vi "SALVAR.vi"() -> ()   [LabVIEW 2014]
uses:
  Global 5.vi
  Global 2.vi
  <vilib>/Utility/file.llb/Write To Spreadsheet File (DBL).vi
panel:
  out "Elapsed Time (s)":dbl
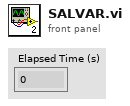
[diagram p1: front panel]
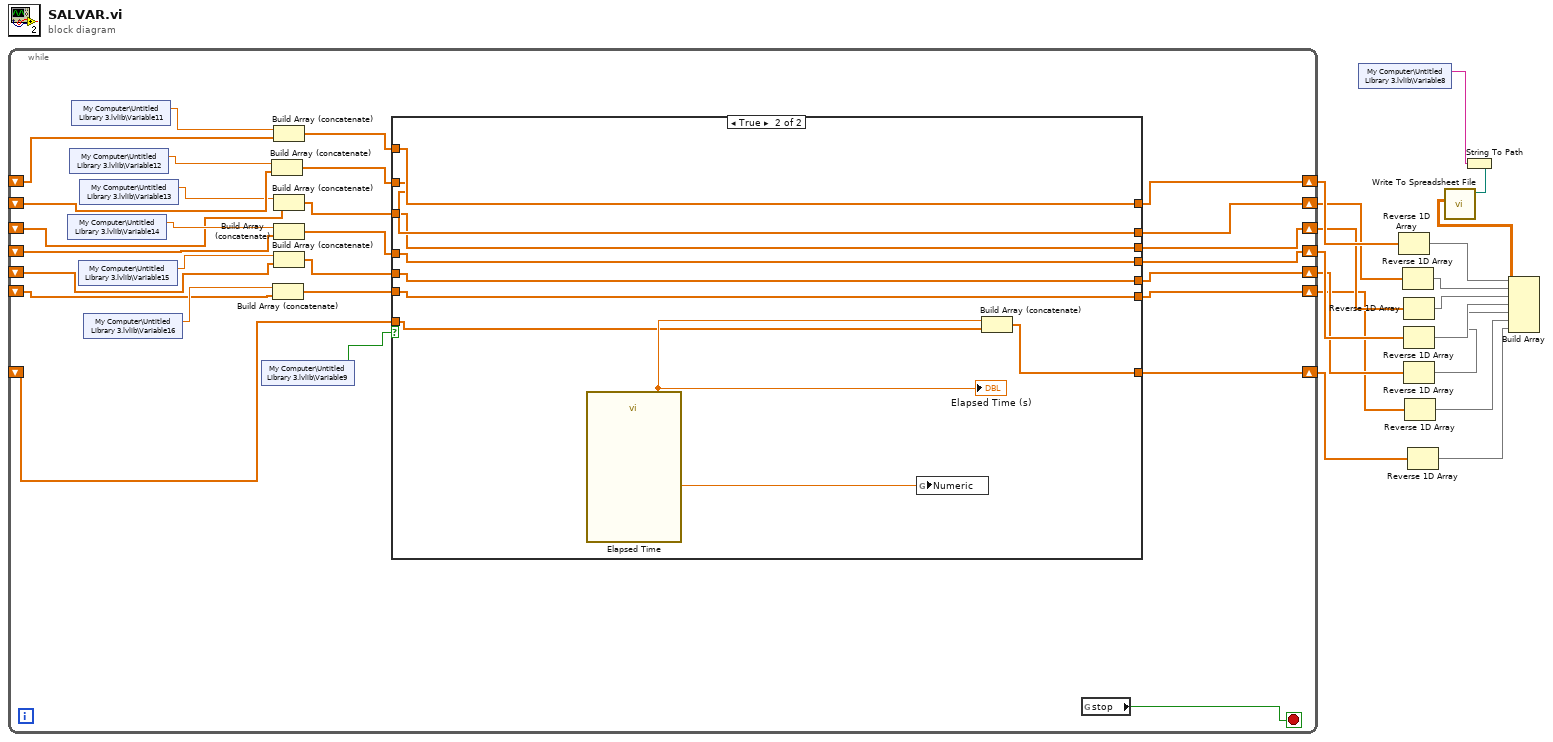
[diagram p0: block diagram]
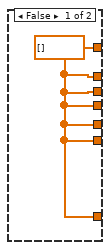
[diagram p2: hidden frame]
diagram:
  n1 = while {
    shift-right: [w42] -> w8
    shift-left: _ -> [w43]
    shift-right: [w23] -> w6
    shift-left: _ -> [w40]
    shift-right: [w22] -> w5
    shift-left: _ -> [w38]
    shift-right: [w21] -> w4
    shift-left: _ -> [w27]
    shift-right: [w20] -> w3
    shift-left: _ -> [w26]
    shift-right: [w19] -> w2
    shift-left: _ -> [w25]
    shift-right: [w18] -> w1
    shift-left: _ -> [w24]
    stop <- w45 stop-if-true
    n2 = shared-variable "My Computer\\Untitled Library 3.lvlib\\Variable14"() -> (w34:dbl)  [unwired: 1 in, 1 out]
    n3 = shared-variable "My Computer\\Untitled Library 3.lvlib\\Variable12"() -> (w39:dbl)  [unwired: 1 in, 1 out]
    n4 = shared-variable "My Computer\\Untitled Library 3.lvlib\\Variable11"() -> (w41:dbl)  [unwired: 1 in, 1 out]
    n5 = shared-variable "My Computer\\Untitled Library 3.lvlib\\Variable15"() -> (w33:dbl)  [unwired: 1 in, 1 out]
    n6 = shared-variable "My Computer\\Untitled Library 3.lvlib\\Variable13"() -> (w35:dbl)  [unwired: 1 in, 1 out]
    n7 = shared-variable "My Computer\\Untitled Library 3.lvlib\\Variable16"() -> (w32:dbl)  [unwired: 1 in, 1 out]
    n8 = shared-variable "My Computer\\Untitled Library 3.lvlib\\Variable9"() -> (w44:bool)  [unwired: 1 in, 1 out]
    n9 = Build Array (concatenate)(w39, w38) -> (w36:dbl[])
    n10 = Build Array (concatenate)(w32, w24) -> (w28:dbl[])
    n11 = Build Array (concatenate)(w41, w40) -> (w37:dbl[])
    n12 = Build Array (concatenate)(w35, w27) -> (w31:dbl[])
    n13 = Build Array (concatenate)(w34, w26) -> (w30:dbl[])
    n14 = Build Array (concatenate)(w33, w25) -> (w29:dbl[])
    n15 = case shown="True" w44 {
      tunnel: [w46 w53] -> w42
      tunnel: w43 -> [_ w54]
      tunnel: [w46 w52] -> w23
      tunnel: w37 -> [_ w52]
      tunnel: w36 -> [_ w51]
      tunnel: [w46 w51] -> w22
      tunnel: w31 -> [_ w50]
      tunnel: [w46 w50] -> w21
      tunnel: w30 -> [_ w49]
      tunnel: [w46 w49] -> w20
      tunnel: w29 -> [_ w48]
      tunnel: [w46 w48] -> w19
      tunnel: w28 -> [_ w47]
      tunnel: [w46 w47] -> w18
      frame False {
        w46 = dbl[] []
      }
      frame True {
        n16 = call "Elapsed Time"() -> ("Elapsed Time (s)"=w55:dbl)  [unwired: 12 in, 7 out]
        "Elapsed Time (s)" <- w55
        n17 = global write "Global 2.vi" "Numeric"(w55) -> ()
        n18 = Build Array (concatenate)(w55, w54) -> (w53:dbl[])
      }
    }
    n19 = global read "Global 5.vi" "stop"() -> (w45:bool)
  }
  n20 = shared-variable "My Computer\\Untitled Library 3.lvlib\\Variable8"() -> (w16:string)  [unwired: 1 in, 1 out]
  n21 = Reverse 1D Array(array=w6) -> (reversed array=w15:dbl[])
  n22 = Reverse 1D Array(array=w5) -> (reversed array=w14:dbl[])
  n23 = Reverse 1D Array(array=w4) -> (reversed array=w13:dbl[])
  n24 = Reverse 1D Array(array=w3) -> (reversed array=w12:dbl[])
  n25 = Reverse 1D Array(array=w2) -> (reversed array=w11:dbl[])
  n26 = Reverse 1D Array(array=w1) -> (reversed array=w9:dbl[])
  n27 = Reverse 1D Array(array=w8) -> (reversed array=w7:dbl[])
  n28 = String To Path(string=w16) -> (path=w17:path)
  n29 = Build Array(w15, w14, w13, w12, w11, w9, w7) -> (w10:dbl[][])
  n30 = call-poly <vilib>:"Write To Spreadsheet File.vi"("2D data"=w10, "file path (dialog if empty)"=w17) -> ()  [unwired: 6 in, 1 out]
